vi "TestFileMgr1.vi"() -> ()   [LabVIEW 2017]
uses:
  <vilib>/addons/Qbus/Qbus.lvclass
  <vilib>/addons/InsightCM/Devices/Shared/Common/ServerComm/ServerComm.lvlib
  <vilib>/NI/Software Watchdog/Pound/Pound.lvclass
  <vilib>/addons/InsightCM/Devices/Shared/Common/FileManager/FileManager.lvlib
  <vilib>/addons/InsightCM/Devices/Shared/FileManager/controls/SendFileRoutedMessage.ctl
  <vilib>/addons/TimerProcess/TimerProcess.lvlib
  <vilib>/addons/InsightCM/MessageBus/Base/controls/ConnectionInfo.ctl
panel:
  in  "Path":path
  in  "SendFile":bool
  out "Listbox":i32(listbox)
  in  "stop":bool
  in  "ConnInfo":T1={"ClientName"="Test4", "TransceiverHost"="10.2.64.59", "TransceiverPort"=6342, "Password"="password"}
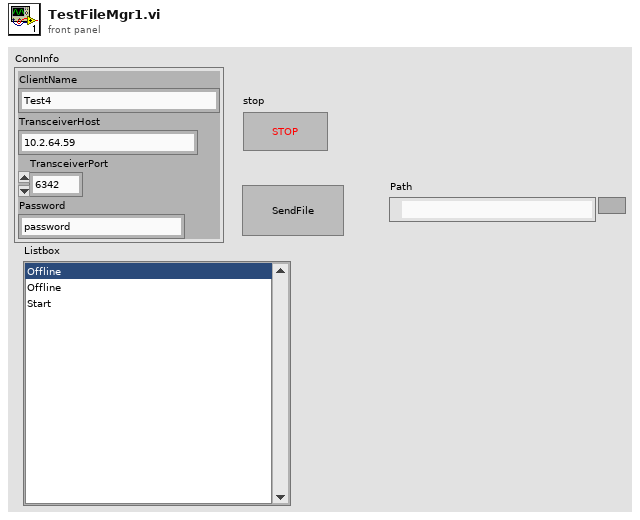
[diagram p1: front panel]
types:
  T1 = typedef "ConnectionInfo.ctl" = cluster{"ClientName":string, "TransceiverHost":string, "TransceiverPort":u16, "Password":string}
  T2 = typedef "FileManager.lvlib/SendFileRoutedMessage.ctl" = cluster{"Filepath":path, "DataGroup":string, "OperatingState":string, "Copy":bool, "StreamId":string, "LastBlock":bool}
  T3 = typedef "ServerComm.lvlib/ConnectionStatus.ctl" = enum16{"Offline", "NotAuthorized", "Online"}
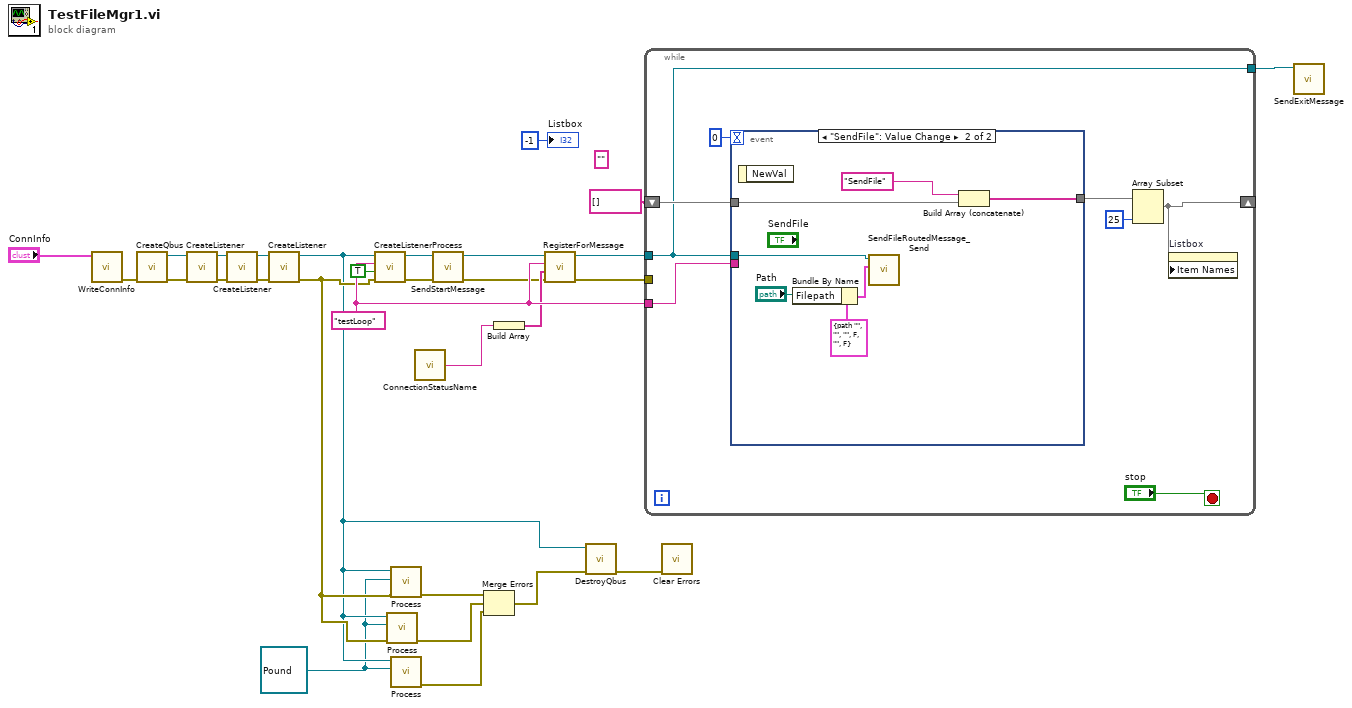
[diagram p0: block diagram]
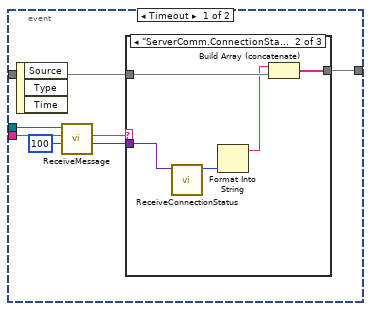
[diagram p2: hidden frame]
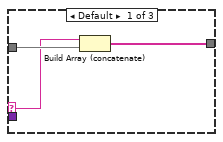
[diagram p3: hidden frame]
diagram:
  (unwired) ""
  w5 = refnum<class "Pound.lvclass"> refnum ("Pound in")
  w19 = "testLoop" ("ProcessName")
  n1 = call <vilib>:"WriteConnInfo.vi"("connection info"="ConnInfo") -> ("error out"=w24:errorcluster)  [unwired: 10 in]
  n2 = call <vilib>:"CreateQbus.vi"("error in (no error)"=w24) -> ("error out"=w14:errorcluster, "Qbus"=w15:refnum<class "Qbus.lvclass">)  [unwired: 9 in]
  n3 = call <vilib>:"CreateListener.vi"("error in (no error)"=w14, "Qbus in"=w15) -> ("error out"=w3:errorcluster, "Qbus out"=w4:refnum<class "Qbus.lvclass">)  [unwired: 8 in]
  n4 = call <vilib>:"CreateListener.vi"("error in (no error)"=w3, "qbus in"=w4) -> ("error out"=w2:errorcluster, "qbus out"=w1:refnum<class "Qbus.lvclass">)  [unwired: 8 in]
  n5 = call <vilib>:"CreateListener.vi"("error in (no error)"=w2, "Qbus in"=w1) -> ("error out"=w8:errorcluster, "Qbus out"=w6:refnum<class "Qbus.lvclass">)  [unwired: 8 in]
  n6 = call <vilib>:"CreateListenerProcess.vi"("error in (no error)"=w8, "master"=TRUE ("Master"), "process name"=w19, "Qbus in"=w6) -> ("error in (no error)"=w28:errorcluster, "Qbus out"=w29:refnum<class "Qbus.lvclass">)  [unwired: 6 in]
  n7 = call <vilib>:"Process.vi"("error in (no error)"=w8, "Pound in"=w5, "Qbus in"=w6) -> ("error out"=w25:errorcluster)  [unwired: 8 in]
  n8 = call <vilib>:"Process.vi"("error in (no error)"=w8, "pound in"=w5, "qbus in"=w6) -> ("error out"=w7:errorcluster)  [unwired: 8 in]
  n9 = call <vilib>:"Process.vi"("Pound in"=w5, "Qbus in"=w6) -> ("error out"=w13:errorcluster)  [unwired: 9 in]
  n10 = call <vilib>:"ConnectionStatusName.vi"() -> ("message name"=w16:string)  [unwired: 5 in]
  n11 = call <vilib>:"SendStartMessage.vi"("error in (no error)"=w28, "Qbus in"=w29) -> ("error in (no error)"=w10:errorcluster, "Qbus out"=w9:refnum<class "Qbus.lvclass">)  [unwired: 8 in]
  n12 = Merge Errors(w7, w25, w13) -> (w26:errorcluster)
  n13 = Build Array(w16) -> (w18:string[])
  n14 = call <vilib>:"RegisterForMessage.vi"("error in (no error)"=w10, "message names"=w18, "process name"=w19, "Qbus in"=w9) -> ("error in (no error)"=w11:errorcluster, "Qbus out"=w12:refnum<class "Qbus.lvclass">)  [unwired: 6 in]
  n15 = call <vilib>:"DestroyQbus.vi"("error in (no error)"=w26, "Qbus"=w6) -> ("error in (no error)"=w20:errorcluster)  [unwired: 9 in]
  n16 = while {
    tunnel: w12 -> [w31]
    tunnel: w19 -> [w37]
    tunnel: [w31] -> w22
    shift-right: [w32] -> _
    shift-left: string[] [] -> [w35]
    tunnel: w11 -> [_]
    stop <- "stop" stop-if-true
    n17 = event shown="[1] \"SendFile\": Value Change" {
      selector: _ -> [_ _]
      dyn-events: _ -> [_ _]
      timeout: 0 -> [_ _]
      tunnel: w37 -> [w44 _]
      tunnel: w35 -> [w41 w60]
      tunnel: [w40 w59] -> w33
      tunnel: w31 -> [w38 w57]
      event Timeout {
        n18 = event-data() -> ()  [unwired: 1 in, 3 out]
        n19 = call <vilib>:"ReceiveMessage.vi"("timeout (0)"=100, "process name"=w44, "Qbus in"=w38) -> ("message value"=w39:variant, "message name"=w42:string)  [unwired: 3 in, 4 out]
        n20 = case shown="\"ServerComm.ConnectionStatus\"" w42 {
          selector: w42 -> [w46 _ _]
          tunnel: [w45 w51 w53] -> w40
          tunnel: w41 -> [w47 w52 w53]
          tunnel: w39 -> [_ w49 _]
          frame Default {
            n21 = Build Array (concatenate)(w46, w47) -> (w45:string[])
          }
          frame "ServerComm.ConnectionStatus" {
            n22 = call <vilib>:"ReceiveConnectionStatus.vi"("body"=w49) -> ("status"=w48:T3)  [unwired: 7 in, 3 out]
            n23 = Format Into String(w48) -> (resulting string=w50:string)  [unwired: 3 in, 1 out]
            n24 = Build Array (concatenate)(w50, w52) -> (w51:string[])
          }
          frame "" {
          }
        }
      }
      event "SendFile": Value Change {
        n25 = event-data() -> ()  [unwired: 1 in, 1 out]
        n26 = Bundle By Name(cluster=T2 {"Filepath"=path "", "DataGroup"="", "OperatingState"="", "Copy"=FALSE, "StreamId"="", "LastBlock"=FALSE} ("send file"), "Filepath"="Path") -> (w55:T2)
        n27 = call <vilib>:"SendFileRoutedMessage_Send.vi"("send file"=w55, "Qbus in"=w57) -> ()  [unwired: 8 in, 2 out]
        n28 = Build Array (concatenate)("SendFile", w60) -> (w59:string[])
      }
    }
    n29 = Array Subset(array=w33, length=25) -> (w32:string[])  [unwired: 1 in]
    n30 = property on="Listbox" class="LstBox (strict)"("Item Names"=w32) -> ()  [unwired: 2 in, 2 out]
  }
  n31 = call <vilib>:"Clear Errors.vi"("error in (no error)"=w20) -> ()  [unwired: 5 in, 2 out]
  n32 = call <vilib>:"SendExitMessage.vi"("Qbus in"=w22) -> ()  [unwired: 9 in, 2 out]
  "Listbox" <- -1 ("Listbox")
